vi "Autonomous Independent.vi"   [LabVIEW 2012]
doc: "This VI is called when autonomous begins, and will automatically be terminated when autonomous ends. You can carry out timed or sensor driven robot movement independently without needing to return to the caller."
uses:
  shooter states.ctl
  <vilib>/Rock Robotics/WPI/Relay/WPI_RelayValue.ctl
  Robot Global Data.vi
  <vilib>/Rock Robotics/WPI/Joystick/WPI_JoystickGetSetRefNum.vi
types:
  T1 = typedef "shooter states.ctl" = enum16{"init", "shooter", "feed", "stop 1", "feed 2", "stop 2", "feed 3", "stop"}
  T2 = typedef "WPI_JoystickDevRef.ctl" = cluster{"Device":T3}
  T3 = typedef "WPI_JoystickDeviceEnum.ctl" = enum16{"USB 1", "USB 2", "USB 3", "USB 4", "Kinect 1", "Kinect 2"}
  T4 = cluster{"axis 1 (x)":dbl, "axis 2 (y)":dbl, "axis 3 (throttle)":dbl, "axis 4":dbl, "axis 5":dbl, "axis 6":dbl}
  T5 = typedef "WPI_MotorControlDeviceRef.ctl" = cluster{"DeviceStatus":errorcluster, "Type":enum16{"PWM", "CAN"}, "PWM":cluster{"Digital Module":T6, "PWM Channel":T7, "DeadBand":T8}, "CAN":cluster{"Device Number":u8, "Control Mode":T9, "Semaphore":T10, "Max Vout":dbl}, "Invert":bool, "TransformRef":T11, "InvTransformRef":T11}
  T6 = typedef "FPGA_TypedefDigitalModule.ctl" = enum16{"Digital Module 1", "Digital Module 2"}
  T7 = typedef "FPGA_DIOPWMChannel.ctl" = enum8{"PWM 1", "PWM 2", "PWM 3", "PWM 4", "PWM 5", "PWM 6", "PWM 7", "PWM 8", "PWM 9", "PWM 10", "Invalid"}
  T8 = typedef "WPI_PWMDeadband.ctl" = cluster{"Name":string, "maxPositivePwm":i32, "minPositivePwm":i32, "centerPwm":i32, "maxNegativePwm":i32, "minNegativePwm":i32, "angularRange":u16}
  T9 = typedef "WPI_CANJaguar_ControlMode.ctl" = enum8{"Percent VBus", "Current", "Speed", "Position", "Voltage"}
  T10 = typedef "Semaphore RefNum" = refnum<k1>
  T11 = typedef "WPI_PWMTransform_ConPane.ctl" = refnum<vi>
  T12 = typedef "WPI_RelayDevRef.ctl" = cluster{"DevStatus":errorcluster, "Relay Channel":T13, "Digital Module":T6, "Relay Direction":T14}
  T13 = typedef "FPGA_DIORelayChannel.ctl" = enum8{"Relay 1", "Relay 2", "Relay 3", "Relay 4", "Relay 5", "Relay 6", "Relay 7", "Relay 8", "Invalid"}
  T14 = typedef "WPI_RelayDirection.ctl" = enum16{"Both directions", "Forward only", "Reverse only"}
  T15 = typedef "WPI_DigitalInputDevRef.ctl" = cluster{"DevStatus":errorcluster, "DIO Channel":T16, "Digital Module":T6}
  T16 = typedef "FPGA_DIOChannel.ctl" = enum8{"DIO 1", "DIO 2", "DIO 3", "DIO 4", "DIO 5", "DIO 6", "DIO 7", "DIO 8", "DIO 9", "DIO 10", "DIO 11", "DIO 12", "DIO 13", "DIO 14", "Invalid"}
  T17 = typedef "WPI_RelayValue.ctl" = enum16{"Off", "On", "Forward", "Reverse"}
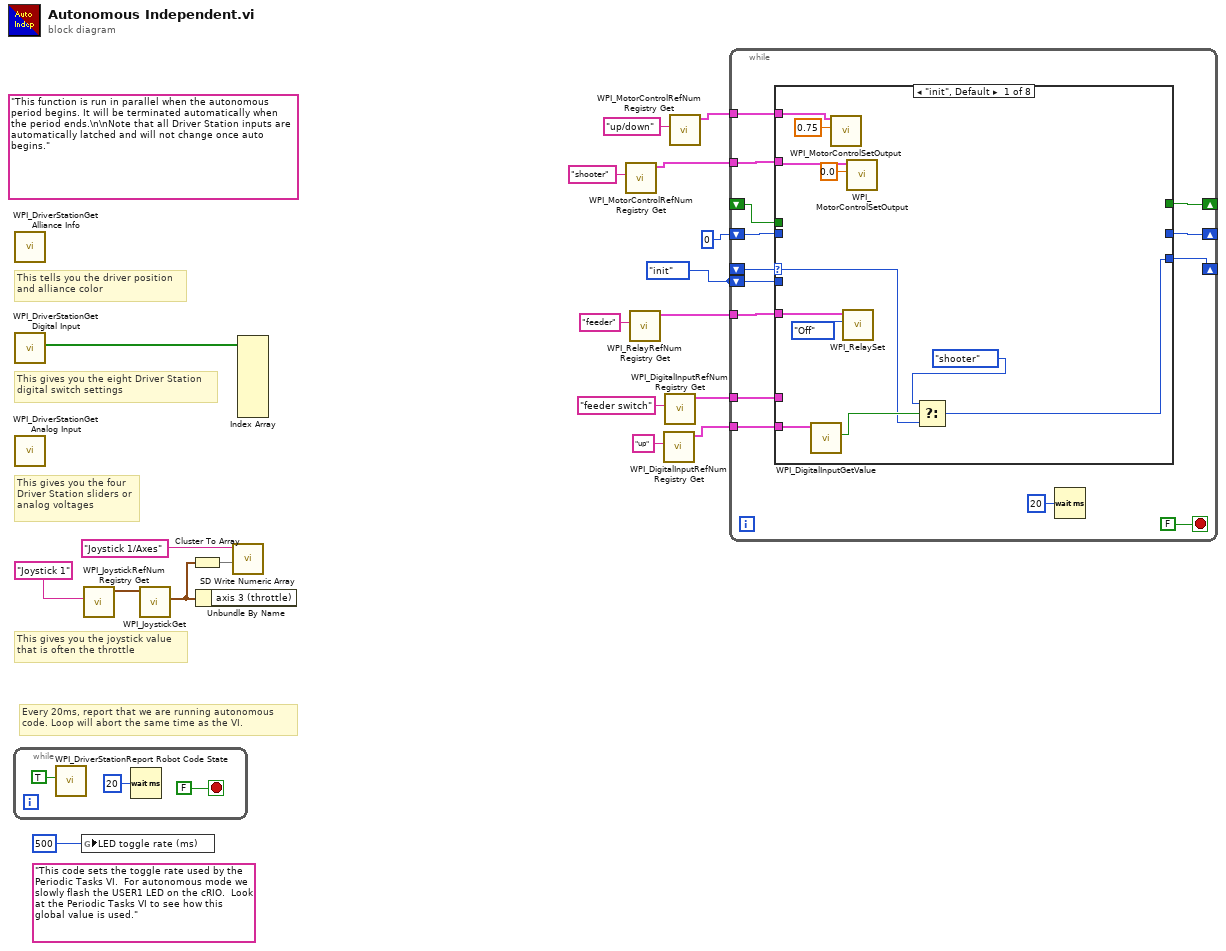
[diagram p0: block diagram]
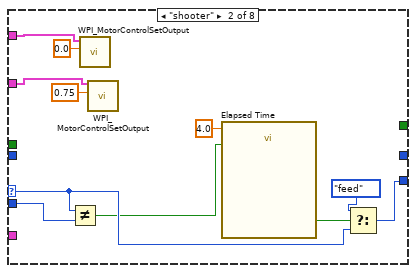
[diagram p2: hidden frame]
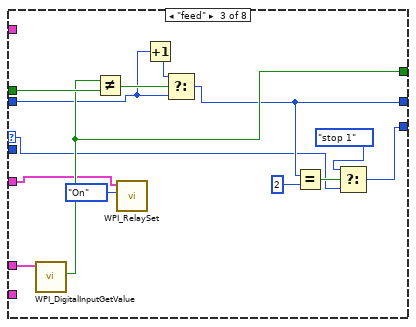
[diagram p3: hidden frame]
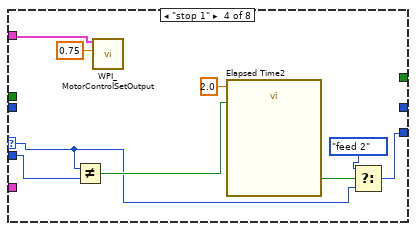
[diagram p4: hidden frame]
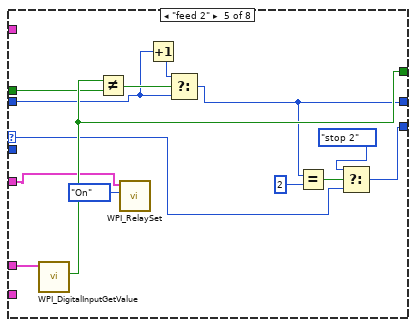
[diagram p5: hidden frame]
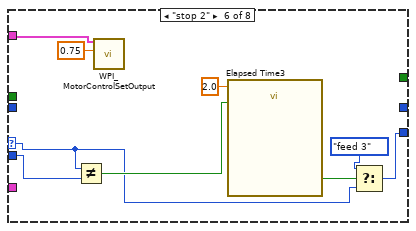
[diagram p6: hidden frame]
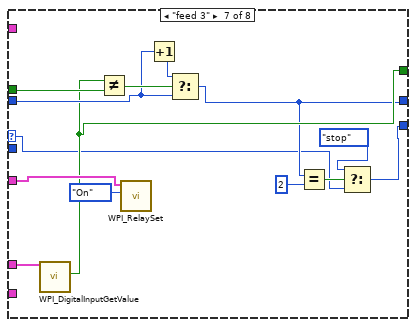
[diagram p7: hidden frame]
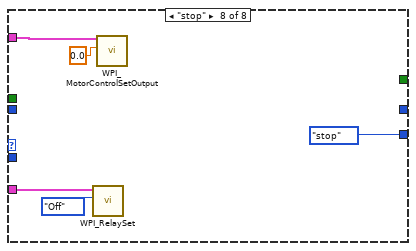
[diagram p8: hidden frame]
diagram:
  w6 = shooter_states."init"
  (unwired) "This code sets the toggle rate used by the Periodic Tasks VI.  For autonomous mode we slowly flash the USER1 LED on the cRIO.  Look at the Periodic Tasks VI to see how this global value is used."
  (unwired) "This function is run in parallel when the autonomous period begins. It will be terminated automatically when the period ends.\n\nNote that all Driver Station inputs are automatically latched and will not change once auto begins."
  # "Every 20ms, report that we are running autonomous\ncode. Loop will abort the same time as the VI."
  # "This gives you the joystick value\nthat is often the throttle"
  # "This tells you the driver position\nand alliance color"
  # "This gives you the eight Driver Station\ndigital switch settings"
  # "This gives you the four\nDriver Station sliders or\nanalog voltages"
  n1 = while {
    stop <- FALSE stop-if-true
    n2 = call <vilib>:"WPI_DriverStationReport Robot Code State.vi"("Autonomous"=TRUE) -> ()  [unwired: 10 in, 1 out]
    n3 = Wait (ms)(milliseconds to wait=u32 20) -> ()  [unwired: 1 out]
  }
  n4 = call <vilib>:"WPI_DriverStationGet Alliance Info.vi"() -> ()  [unwired: 12 out]
  n5 = call <vilib>:"WPI_DriverStationGet Digital Input.vi"() -> ("Driver Station Digital Input (1-8)"=w19:bool[])  [unwired: 11 out]
  n6 = call <vilib>:"WPI_DriverStationGet Analog Input.vi"() -> ()  [unwired: 12 out]
  n7 = global write "Robot Global Data.vi" "LED toggle rate (ms)"(u32 500 ("LED ms toggle rate")) -> ()
  n8 = call <vilib>:"WPI_JoystickRefNum Registry Get.vi"("refnum name"="Joystick 1") -> ("JoystickDevRef"=w17:T2)  [unwired: 1 in, 9 out]
  n9 = call <vilib>:"WPI_JoystickGet.vi"("JoystickDevRef"=w17) -> ("Axes"=w14:T4)  [unwired: 1 in, 5 out]
  n10 = Cluster To Array(cluster=w14) -> (array=w15:dbl[])
  n11 = Unbundle By Name(w14) -> ()  [unwired: 1 out]
  n12 = call <vilib>:"SD Write Numeric Array.vi"("Numeric Array"=w15, "Name"="Joystick 1/Axes") -> ()  [unwired: 8 in, 2 out]
  n13 = Index Array(array=w19) -> ()  [unwired: 8 in, 8 out]
  n14 = call <vilib>:"WPI_MotorControlRefNum Registry Get.vi"("refnum name"="shooter") -> ("MotorControlDevRef"=w11:T5)  [unwired: 9 in, 1 out]
  n15 = call <vilib>:"WPI_RelayRefNum Registry Get.vi"("refnum name"="feeder") -> ("RelayDevRef"=w9:T12)  [unwired: 9 in, 1 out]
  n16 = call <vilib>:"WPI_DigitalInputRefNum Registry Get.vi"("refnum name"="up") -> ("DigitalInputDevRef"=w3:T15)  [unwired: 9 in, 1 out]
  n17 = call <vilib>:"WPI_DigitalInputRefNum Registry Get.vi"("refnum name"="feeder switch") -> ("DigitalInputDevRef"=w7:T15)  [unwired: 9 in, 1 out]
  n18 = call <vilib>:"WPI_MotorControlRefNum Registry Get.vi"("refnum name"="up/down") -> ("MotorControlDevRef"=w1:T5)  [unwired: 9 in, 1 out]
  n19 = while {
    tunnel: w11 -> [w33]
    tunnel: w9 -> [w32]
    shift-right: [w31] -> _
    shift-left: w6 -> [w34]
    shift-left: w6 -> [w25]
    tunnel: w7 -> [w30]
    shift-right: [w28] -> _
    shift-left: _ -> [w29]
    shift-right: [w26] -> _
    shift-left: 0 -> [w27]
    tunnel: w3 -> [w24]
    tunnel: w1 -> [w23]
    stop <- FALSE stop-if-true
    n20 = case shown="\"init\", Default" w34 {
      selector: w34 -> [w41 w53 w62 w75 w83 w98 w106 _]
      tunnel: w33 -> [w47 w57 _ w76 _ w99 _ w121]
      tunnel: w32 -> [w45 _ w60 _ w86 _ w110 w120]
      tunnel: [w37 w51 w61 w74 w85 w97 w107 shooter_states."stop"] -> w31
      tunnel: w30 -> [_ _ w72 _ w82 _ w105 _]
      tunnel: w29 -> [_ _ w71 _ w88 _ w112 _]
      tunnel: [_ _ w70 _ w89 _ w109 _] -> w28
      tunnel: w27 -> [_ _ w67 _ w87 _ w111 _]
      tunnel: [_ _ w66 _ w84 _ w108 _] -> w26
      tunnel: w25 -> [_ w50 _ w73 _ w96 _ _]
      tunnel: w24 -> [w43 _ _ _ _ _ _ _]
      tunnel: w23 -> [w38 w48 _ _ _ _ _ _]
      frame "init", Default {
        n21 = call <vilib>:"WPI_DigitalInputGetValue.vi"("DigitalInputDevRef"=w43) -> ("Value"=w42:bool)  [unwired: 8 in, 2 out]
        n22 = call <vilib>:"WPI_MotorControlSetOutput.vi"("Output"=0.75, "MotorControlDevRef"=w38) -> ()  [unwired: 7 in, 3 out]
        n23 = call <vilib>:"WPI_RelaySet.vi"("RelayValue"=WPI_RelayValue."Off", "RelayDevRef"=w45) -> ()  [unwired: 8 in, 2 out]
        n24 = call <vilib>:"WPI_MotorControlSetOutput.vi"("Output"=0.0, "MotorControlDevRef"=w47) -> ()  [unwired: 7 in, 3 out]
        n25 = Select(t=shooter_states."shooter", s=w42, f=w41) -> (s? t:f=w37:T1)
      }
      frame "shooter" {
        n26 = Not Equal?(x=w53, y=w50) -> (x != y?=w52:bool)
        n27 = call <vilib>:"WPI_MotorControlSetOutput.vi"("Output"=0.0, "MotorControlDevRef"=w48) -> ()  [unwired: 7 in, 3 out]
        n28 = call <vilib>:"WPI_MotorControlSetOutput.vi"("Output"=0.75, "MotorControlDevRef"=w57) -> ()  [unwired: 7 in, 3 out]
        n29 = call "Elapsed Time"("Time Target (s)"=4.0, "Reset"=w52) -> ("Time has Elapsed"=w55:bool)  [unwired: 10 in, 7 out]
        n30 = Select(t=shooter_states."feed", s=w55, f=w53) -> (s? t:f=w51:T1)
      }
      frame "feed" {
        n31 = call <vilib>:"WPI_DigitalInputGetValue.vi"("DigitalInputDevRef"=w72) -> ("Value"=w70:bool)  [unwired: 8 in, 2 out]
        n32 = Not Equal?(x=w70, y=w71) -> (x != y?=w69:bool)
        n33 = call <vilib>:"WPI_RelaySet.vi"("RelayValue"=WPI_RelayValue."On", "RelayDevRef"=w60) -> ()  [unwired: 8 in, 2 out]
        n34 = Increment(x=w67) -> (x+1=w68:i32)
        n35 = Select(t=w68, s=w69, f=w67) -> (s? t:f=w66:i32)
        n36 = Equal?(x=w66, y=2) -> (x = y?=w64:bool)
        n37 = Select(t=shooter_states."stop 1", s=w64, f=w62) -> (s? t:f=w61:T1)
      }
      frame "stop 1" {
        n38 = Not Equal?(x=w75, y=w73) -> (x != y?=w77:bool)
        n39 = call <vilib>:"WPI_MotorControlSetOutput.vi"("Output"=0.75, "MotorControlDevRef"=w76) -> ()  [unwired: 7 in, 3 out]
        n40 = call "Elapsed Time2"("Time Target (s)"=2.0, "Reset"=w77) -> ("Time has Elapsed"=w79:bool)  [unwired: 10 in, 7 out]
        n41 = Select(t=shooter_states."feed 2", s=w79, f=w75) -> (s? t:f=w74:T1)
      }
      frame "feed 2" {
        n42 = call <vilib>:"WPI_DigitalInputGetValue.vi"("DigitalInputDevRef"=w82) -> ("Value"=w89:bool)  [unwired: 8 in, 2 out]
        n43 = Not Equal?(x=w89, y=w88) -> (x != y?=w95:bool)
        n44 = call <vilib>:"WPI_RelaySet.vi"("RelayValue"=WPI_RelayValue."On", "RelayDevRef"=w86) -> ()  [unwired: 8 in, 2 out]
        n45 = Increment(x=w87) -> (x+1=w94:i32)
        n46 = Select(t=w94, s=w95, f=w87) -> (s? t:f=w84:i32)
        n47 = Equal?(x=w84, y=2) -> (x = y?=w92:bool)
        n48 = Select(t=shooter_states."stop 2", s=w92, f=w83) -> (s? t:f=w85:T1)
      }
      frame "stop 2" {
        n49 = Not Equal?(x=w98, y=w96) -> (x != y?=w100:bool)
        n50 = call <vilib>:"WPI_MotorControlSetOutput.vi"("Output"=0.75, "MotorControlDevRef"=w99) -> ()  [unwired: 7 in, 3 out]
        n51 = call "Elapsed Time3"("Time Target (s)"=2.0, "Reset"=w100) -> ("Time has Elapsed"=w102:bool)  [unwired: 10 in, 7 out]
        n52 = Select(t=shooter_states."feed 3", s=w102, f=w98) -> (s? t:f=w97:T1)
      }
      frame "feed 3" {
        n53 = call <vilib>:"WPI_DigitalInputGetValue.vi"("DigitalInputDevRef"=w105) -> ("Value"=w109:bool)  [unwired: 8 in, 2 out]
        n54 = Not Equal?(x=w109, y=w112) -> (x != y?=w118:bool)
        n55 = call <vilib>:"WPI_RelaySet.vi"("RelayValue"=WPI_RelayValue."On", "RelayDevRef"=w110) -> ()  [unwired: 8 in, 2 out]
        n56 = Increment(x=w111) -> (x+1=w117:i32)
        n57 = Select(t=w117, s=w118, f=w111) -> (s? t:f=w108:i32)
        n58 = Equal?(x=w108, y=2) -> (x = y?=w115:bool)
        n59 = Select(t=shooter_states."stop", s=w115, f=w106) -> (s? t:f=w107:T1)
      }
      frame "stop" {
        n60 = call <vilib>:"WPI_RelaySet.vi"("RelayValue"=WPI_RelayValue."Off", "RelayDevRef"=w120) -> ()  [unwired: 8 in, 2 out]
        n61 = call <vilib>:"WPI_MotorControlSetOutput.vi"("Output"=0.0, "MotorControlDevRef"=w121) -> ()  [unwired: 7 in, 3 out]
      }
    }
    n62 = Wait (ms)(milliseconds to wait=u32 20) -> ()  [unwired: 1 out]
  }
